vi "Math-Column Sum (CDB).vi"(1 "2D Array":cdb[][](array[numeric])) -> (0 "Column sums":cdb[](array[numeric]))   [LabVIEW 2015]
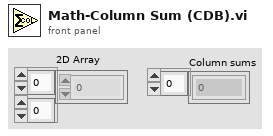
[diagram p1: front panel]
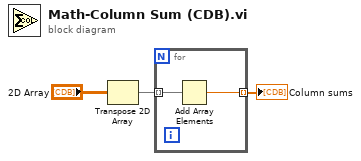
[diagram p0: block diagram]
diagram:
  n1 = Transpose 2D Array(2D array="2D Array") -> (transposed array=w2:cdb[][])
  n2 = for {
    tunnel: w2 -> [w5] mode=indexing
    tunnel: [w4] -> w1 mode=indexing
    n3 = Add Array Elements(numeric array=w5) -> (sum=w4:cdb)
  }
  "Column sums" <- w1
